vi "BuildParamSheet.vi"(2 "StartParamIndices":i32[](array[numeric])=[0, 1, 2, 3, 4, 7, 11, 14, 16, 17, 19], 3 "Params list":string[][](array[string])=[["ADC", "state (0,1,2)", "txt", "C:\\CuspControl\\GPIB and Network\\Cusp\\ADCState.txt", "", ""], ["Camera", "state (0,1)", "txt", "C:\\CuspControl\\GPIB and Network\\Cusp\\CameraState.txt", "", ""], ["Slave", "state (0,1)", "txt", "C:\\CuspControl\\GPIB and Network\\Cusp\\SlaveState.txt", "", ""], ["Wait", "inbit (0...7)", "dac", "0.1", "-1", "-1"], ["e-", "enable (0,1)", "txt", "C:\\CuspControl\\GPIB and Network\\Cusp\\esourceRampVoltandState.txt", "", ""], ["e-", "burn time (s)", "txt", "C:\\CuspControl\\GPIB and Network\\Cusp\\esourceRampVoltandState.txt", "", ""], ["e-", "filament (A)", "txt", "C:\\CuspControl\\GPIB and Network\\Cusp\\esourceRampVoltandState.txt", "", ""], ["RW", "enable (0,1)", "txt", "C:\\CuspControl\\GPIB and Network\\Cusp\\RWparams.txt", "", ""], ["RW", "frequency (Hz)", "txt", "C:\\CuspControl\\GPIB and Network\\Cusp\\RWparams.txt", "", ""], ["RW", "amplitude (V)", "txt", "C:\\CuspControl\\GPIB and Network\\Cusp\\RWparams.txt", "", ""], ["RW", "phase dif (deg)", "txt", "C:\\CuspControl\\GPIB and Network\\Cusp\\RWparams.txt", "", ""], ["HVpulse", "enable (0,1)", "dac", "0.1", "ao0", "10"], ["HVpulse", "amplitude (V)", "dac", "0.1", "ao1", "1"], ["HVpulse", "polarity (0=n)", "dac", "0.1", "ao2", "5"], ["HVptime", "delay (s)", "txt", "C:\\CuspControl\\GPIB and Network\\Cusp\\HVPulseTiming.txt", "", ""], ["HVptime", "width (s)", "txt", "C:\\CuspControl\\GPIB and Network\\Cusp\\HVPulseTiming.txt", "", ""], ["Gcoil", "current (A)", "dac", "0.1", "ao4", "0.11"], ["MCP", "front bias (V)", "dac", "4", "ao5", "0.067"], ["MCP", "back bias (V)", "dac", "4", "ao6", "0.0048"], ["MCP", "phos bias (V)", "dac", "4", "ao7", "0.0020"]], 4 "Actions":T1=[{"Toggle"=TRUE, "Open parameter editor"=FALSE, "Open MacroEditor"=FALSE, "Macro path"=path "", "Duration (s)"=0.001, "Parameters"=[{"Status"="ADC", "Name"="state (0,1,2)", "Value"=0.0, "Changed"=FALSE}, {"Status"="Camera", "Name"="state (0,1)", "Value"=1.0, "Changed"=TRUE}, {"Status"="Slave", "Name"="state (0,1)", "Value"=0.0, "Changed"=FALSE}, {"Status"="Wait", "Name"="inbit (0...7)", "Value"=0.0, "Changed"=FALSE}, {"Status"="e-", "Name"="enable (0,1)", "Value"=0.0, "Changed"=FALSE}, {"Status"="e-", "Name"="burn time (s)", "Value"=0.0, "Changed"=FALSE}, {"Status"="e-", "Name"="filament (A)", "Value"=0.0, "Changed"=FALSE}, {"Status"="RW", "Name"="enable (0,1)", "Value"=0.0, "Changed"=FALSE}, {"Status"="RW", "Name"="frequency (Hz)", "Value"=0.0, "Changed"=FALSE}, {"Status"="RW", "Name"="amplitude (V)", "Value"=0.0, "Changed"=FALSE}, {"Status"="RW", "Name"="phase dif (deg)", "Value"=0.0, "Changed"=FALSE}, {"Status"="HVpulse", "Name"="enable (0,1)", "Value"=0.0, "Changed"=FALSE}, {"Status"="HVpulse", "Name"="amplitude (V)", "Value"=0.0, "Changed"=FALSE}, {"Status"="HVpulse", "Name"="polarity (0=n)", "Value"=0.0, "Changed"=FALSE}, {"Status"="HVptime", "Name"="delay (s)", "Value"=0.0, "Changed"=FALSE}, {"Status"="HVptime", "Name"="width (s)", "Value"=0.0, "Changed"=FALSE}, {"Status"="Gcoil", "Name"="current (A)", "Value"=0.0, "Changed"=FALSE}, {"Status"="MCP", "Name"="front bias (V)", "Value"=0.0, "Changed"=FALSE}, {"Status"="MCP", "Name"="back bias (V)", "Value"=0.0, "Changed"=FALSE}, {"Status"="MCP", "Name"="phos bias (V)", "Value"=0.0, "Changed"=FALSE}], "Comment"="", "Reps"=1}, {"Toggle"=TRUE, "Open parameter editor"=FALSE, "Open MacroEditor"=FALSE, "Macro path"=path "", "Duration (s)"=0.011, "Parameters"=[{"Status"="ADC", "Name"="state (0,1,2)", "Value"=0.0, "Changed"=FALSE}, {"Status"="Camera", "Name"="state (0,1)", "Value"=1.0, "Changed"=FALSE}, {"Status"="Slave", "Name"="state (0,1)", "Value"=0.0, "Changed"=FALSE}, {"Status"="Wait", "Name"="inbit (0...7)", "Value"=0.0, "Changed"=FALSE}, {"Status"="e-", "Name"="enable (0,1)", "Value"=0.0, "Changed"=FALSE}, {"Status"="e-", "Name"="burn time (s)", "Value"=0.0, "Changed"=FALSE}, {"Status"="e-", "Name"="filament (A)", "Value"=0.0, "Changed"=FALSE}, {"Status"="RW", "Name"="enable (0,1)", "Value"=0.0, "Changed"=FALSE}, {"Status"="RW", "Name"="frequency (Hz)", "Value"=0.0, "Changed"=FALSE}, {"Status"="RW", "Name"="amplitude (V)", "Value"=0.0, "Changed"=FALSE}, {"Status"="RW", "Name"="phase dif (deg)", "Value"=1.0, "Changed"=TRUE}, {"Status"="HVpulse", "Name"="enable (0,1)", "Value"=0.0, "Changed"=FALSE}, {"Status"="HVpulse", "Name"="amplitude (V)", "Value"=0.0, "Changed"=FALSE}, {"Status"="HVpulse", "Name"="polarity (0=n)", "Value"=0.0, "Changed"=FALSE}, {"Status"="HVptime", "Name"="delay (s)", "Value"=0.0, "Changed"=FALSE}, {"Status"="HVptime", "Name"="width (s)", "Value"=0.0, "Changed"=FALSE}, {"Status"="Gcoil", "Name"="current (A)", "Value"=0.0, "Changed"=FALSE}, {"Status"="MCP", "Name"="front bias (V)", "Value"=0.0, "Changed"=FALSE}, {"Status"="MCP", "Name"="back bias (V)", "Value"=0.0, "Changed"=FALSE}, {"Status"="MCP", "Name"="phos bias (V)", "Value"=0.0, "Changed"=FALSE}], "Comment"="", "Reps"=1}, {"Toggle"=TRUE, "Open parameter editor"=FALSE, "Open MacroEditor"=FALSE, "Macro path"=path "", "Duration (s)"=0.011, "Parameters"=[{"Status"="ADC", "Name"="state (0,1,2)", "Value"=0.0, "Changed"=FALSE}, {"Status"="Camera", "Name"="state (0,1)", "Value"=0.0, "Changed"=TRUE}, {"Status"="Slave", "Name"="state (0,1)", "Value"=0.0, "Changed"=FALSE}, {"Status"="Wait", "Name"="inbit (0...7)", "Value"=0.0, "Changed"=FALSE}, {"Status"="e-", "Name"="enable (0,1)", "Value"=0.0, "Changed"=FALSE}, {"Status"="e-", "Name"="burn time (s)", "Value"=0.0, "Changed"=FALSE}, {"Status"="e-", "Name"="filament (A)", "Value"=0.0, "Changed"=FALSE}, {"Status"="RW", "Name"="enable (0,1)", "Value"=0.0, "Changed"=FALSE}, {"Status"="RW", "Name"="frequency (Hz)", "Value"=0.0, "Changed"=FALSE}, {"Status"="RW", "Name"="amplitude (V)", "Value"=0.0, "Changed"=FALSE}, {"Status"="RW", "Name"="phase dif (deg)", "Value"=2.0, "Changed"=TRUE}, {"Status"="HVpulse", "Name"="enable (0,1)", "Value"=0.0, "Changed"=FALSE}, {"Status"="HVpulse", "Name"="amplitude (V)", "Value"=0.0, "Changed"=FALSE}, {"Status"="HVpulse", "Name"="polarity (0=n)", "Value"=5.0, "Changed"=TRUE}, {"Status"="HVptime", "Name"="delay (s)", "Value"=0.0, "Changed"=FALSE}, {"Status"="HVptime", "Name"="width (s)", "Value"=0.0, "Changed"=FALSE}, {"Status"="Gcoil", "Name"="current (A)", "Value"=3.0, "Changed"=TRUE}, {"Status"="MCP", "Name"="front bias (V)", "Value"=0.0, "Changed"=FALSE}, {"Status"="MCP", "Name"="back bias (V)", "Value"=0.0, "Changed"=FALSE}, {"Status"="MCP", "Name"="phos bias (V)", "Value"=0.0, "Changed"=FALSE}], "Comment"="", "Reps"=1}] {"Reps" min=1 step=1; "Parameters"."Value" format="%_6p"; "Duration (s)" min=0.01 step=0.001 format="%_6p"}) -> (0 "DAC cmds":string[](array[string])=["Action 0\n", "Action 1\n", "Action 2\n0.1\tao0\t10\t0.000000E+0\r\n0.1\tao1\t1\t0.000000E+0\r\n0.1\tao2\t5\t5.000000E+0\r\n0.1\tao4\t0.11\t3.000000E+0\r\n"], 1 "txt cmds":string[](array[string])=["Action 0\nC:\\CuspControl\\GPIB and Network\\Cusp\\CameraState.txt\t1.000000E+0\r\n", "Action 1\nC:\\CuspControl\\GPIB and Network\\Cusp\\RWparams.txt\t0.000000E+0\t0.000000E+0\t0.000000E+0\t1.000000E+0\r\n", "Action 2\nC:\\CuspControl\\GPIB and Network\\Cusp\\CameraState.txt\t0.000000E+0\r\nC:\\CuspControl\\GPIB and Network\\Cusp\\esourceRampVoltandState.txt\t1.000000E+0\t3.000000E+1\t3.000000E-1\r\nC:\\CuspControl\\GPIB and Network\\Cusp\\RWparams.txt\t0.000000E+0\t0.000000E+0\t5.000000E+0\t2.000000E+0\r\n"])   [LabVIEW 2018]
uses:
  QBuilder Files/Actions_arr.ctl
  QBuilder Files/Action.ctl
  QBuilder Files/Parameters.ctl
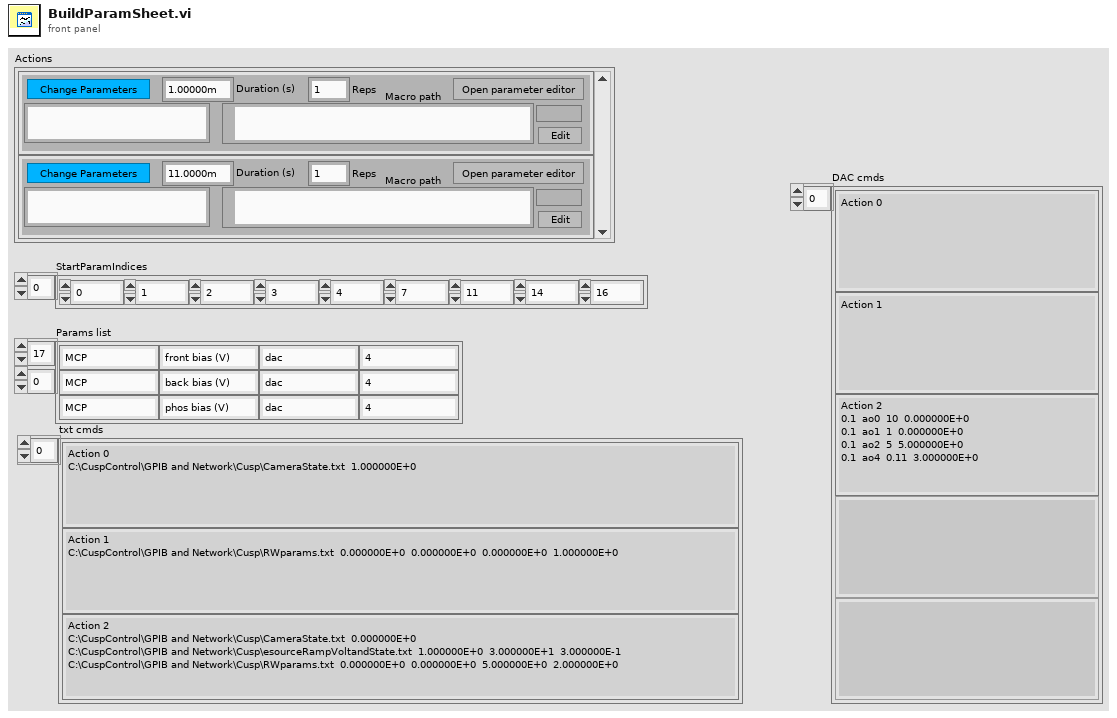
[diagram p1: front panel]
types:
  T1 = typedef "Actions_arr.ctl" = T2[]
  T2 = typedef "Action.ctl" = cluster{"Toggle":bool, "Open parameter editor":bool, "Open MacroEditor":bool, "Macro path":path, "Duration (s)":dbl, "Parameters":T3, "Comment":string, "Reps":i32}
  T3 = typedef "Parameters.ctl" = cluster{"Status":string, "Name":string, "Value":dbl, "Changed":bool}[]
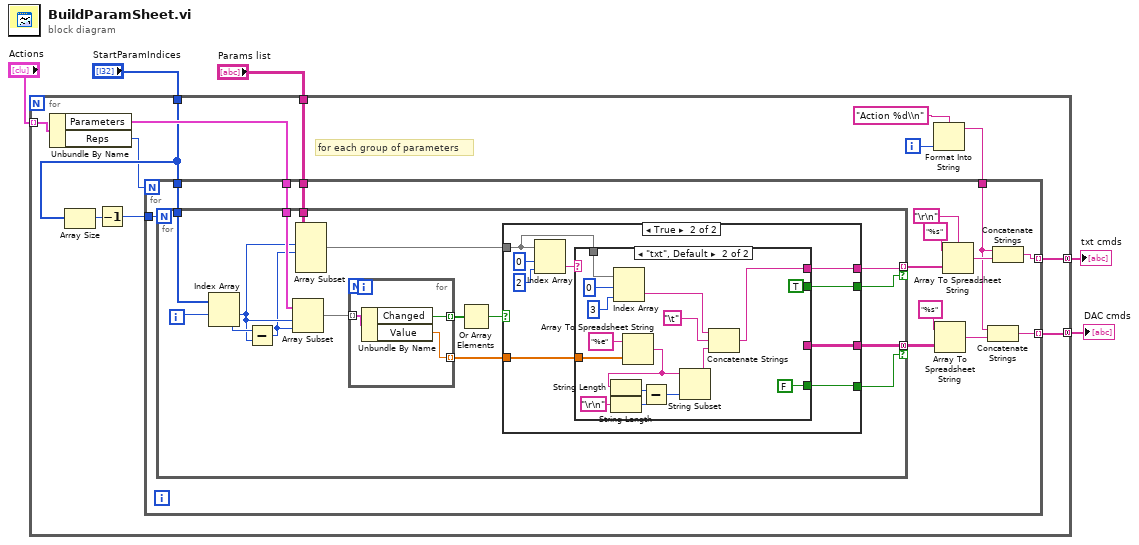
[diagram p0: block diagram]
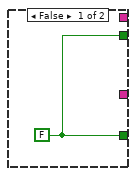
[diagram p2: hidden frame]
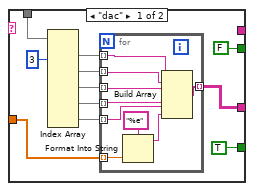
[diagram p3: hidden frame]
diagram:
  n1 = for {
    tunnel: "Actions" -> [w17] mode=indexing
    tunnel: "StartParamIndices" -> [w13]
    tunnel: "Params list" -> [w12]
    tunnel: [w7] -> w2 mode=concatenating
    tunnel: [w8] -> w1 mode=concatenating
    i -> [w11]
    # "for each group of parameters"
    n2 = Unbundle By Name(w17) -> ("Parameters"=w16:T3, "Reps"=w6:i32)
    n3 = Array Size(array=w13) -> (size(s)=w14:i32)
    n4 = Decrement(x=w14) -> (x-1=w15:i32)
    n5 = Format Into String(format string="Action %d\\n" ("initial string"), w11) -> (resulting string=w10:string)  [unwired: 2 in, 1 out]
    n6 = for {
      N: w6 -> [_]
      tunnel: w16 -> [w31]
      tunnel: w15 -> [w30]
      tunnel: w13 -> [w29]
      tunnel: w12 -> [w28]
      tunnel: w10 -> [w21]
      tunnel: [w19] -> w8 mode=indexing
      tunnel: [w18] -> w7 mode=indexing
      n7 = for {
        N: w30 -> [_]
        tunnel: w31 -> [w42]
        tunnel: [w37] -> w27 mode=concatenating if=w34
        tunnel: w29 -> [w36]
        tunnel: w28 -> [w35]
        tunnel: [w33] -> w22 mode=indexing if=w32
        i -> [w47]
        n8 = Index Array(array=w36, index #1=w47) -> (element #1=w41:i32, element #2=w46:i32)  [unwired: 1 in]
        n9 = Subtract(x=w46, y=w41) -> (x-y=w40:i32)
        n10 = Array Subset(array=w42, index=w41, length=w40) -> (w45:T3)
        n11 = Array Subset(array=w35, index (row)=w41, length (row)=w40) -> (w39:string[][])  [unwired: 2 in]
        n12 = for {
          tunnel: w45 -> [w96] mode=indexing
          tunnel: [w95] -> w44 mode=indexing
          tunnel: [w94] -> w38 mode=indexing
          n13 = Unbundle By Name(w96) -> ("Changed"=w95:bool, "Value"=w94:dbl)
        }
        n14 = Or Array Elements(Boolean array=w44) -> (logical OR=w43:bool)
        n15 = case shown="True" w43 {
          tunnel: w39 -> [_ w53]
          tunnel: w38 -> [_ w54]
          tunnel: [_ w52] -> w37
          tunnel: [w48 w51] -> w34
          tunnel: [_ w50] -> w33
          tunnel: [w48 w49] -> w32
          frame False {
            w48 = FALSE
          }
          frame True {
            n16 = Index Array(array=w53, index (row)=0 ("disabled index (row)"), index (col)=2 ("disabled index (col)")) -> (element=w55:string)
            n17 = case shown="\"txt\", Default" w55 {
              tunnel: w54 -> [w66 w89]
              tunnel: w53 -> [w68 w93]
              tunnel: [w62 _] -> w52
              tunnel: [TRUE FALSE] -> w51
              tunnel: [_ w84] -> w50
              tunnel: [FALSE TRUE] -> w49
              frame "dac" {
                n18 = Index Array(array=w68, index (col) #1=3 ("disabled index (col)")) -> (element #1=w63:string[], element #2=w64:string[], element #3=w65:string[], element #4=w59:string[], element #5=w58:string[])  [unwired: 9 in]
                n19 = for {
                  tunnel: w66 -> [w77] mode=indexing
                  tunnel: w65 -> [w75] mode=indexing
                  tunnel: w64 -> [w74] mode=indexing
                  tunnel: w63 -> [w73] mode=indexing
                  tunnel: [w72] -> w62 mode=indexing
                  tunnel: w59 -> [w71] mode=indexing
                  tunnel: w58 -> [w70] mode=indexing
                  n20 = Format Into String(format string="%e", w77) -> (resulting string=w69:string)  [unwired: 2 in, 1 out]
                  n21 = Build Array(w73, w74, w75, w71, w70, w69) -> (w72:string[])
                }
              }
              frame "txt", Default {
                n22 = String Length(string="\r\n") -> (length=w82:i32)
                n23 = Index Array(array=w93, index (row)=0 ("disabled index (row)"), index (col)=3 ("disabled index (col)")) -> (element=w87:string)
                n24 = Array To Spreadsheet String(array=w89, 3:"%e" ("format string")) -> (spreadsheet string=w83:string)  [unwired: 1 in]
                n25 = String Length(string=w83) -> (length=w81:i32)
                n26 = Subtract(x=w81, y=w82) -> (x-y=w80:i32)
                n27 = String Subset(string=w83, length (rest)=w80) -> (substring=w79:string)  [unwired: 1 in]
                n28 = Concatenate Strings(w87, "\t", w79) -> (w84:string)
              }
            }
          }
        }
      }
      n29 = Array To Spreadsheet String(array=w27, 3:"%s" ("format string")) -> (spreadsheet string=w25:string)  [unwired: 1 in]
      n30 = Array To Spreadsheet String(delimiter (Tab)="\r\n", array=w22, 3:"%s" ("format string")) -> (spreadsheet string=w24:string)
      n31 = Concatenate Strings(w21, w25) -> (w18:string)
      n32 = Concatenate Strings(w21, w24) -> (w19:string)
    }
  }
  "DAC cmds" <- w2
  "txt cmds" <- w1
